vi "FGA Find Client Rec.vi"(3 "Source ID":u32) -> (0 "Record Exists?":bool, 1 "Record out":T1)   [LabVIEW 2011]
uses:
  Source ID Network Location Pair.ctl
  UDP Lib/UDP Network Location.ctl
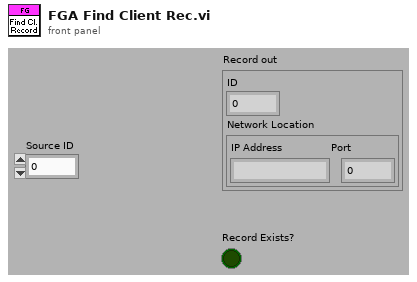
[diagram p1: front panel]
types:
  T1 = typedef "Source ID Network Location Pair.ctl" = cluster{"ID":u32, "Network Location":T2}
  T2 = typedef "UDP Network Location.ctl" = cluster{"IP Address":string, "Port":u16}
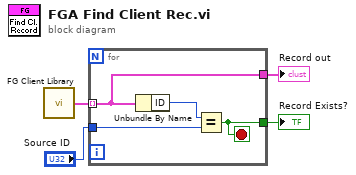
[diagram p0: block diagram]
diagram:
  n1 = call "FG Client Library.vi"() -> ("Client Records out"=w4:T1[])  [unwired: 2 in]
  n2 = for {
    tunnel: w4 -> [w8] mode=indexing
    tunnel: "Source ID" -> [w6]
    tunnel: [w8] -> w2
    tunnel: [w5] -> w1
    stop <- w5 stop-if-true
    n3 = Unbundle By Name(w8) -> ("ID"=w7:u32)
    n4 = Equal?(x=w7, y=w6) -> (x = y?=w5:bool)
  }
  "Record Exists?" <- w1
  "Record out" <- w2
